vi "Rotating_Array.vi"() -> ()   [LabVIEW 2024]
panel:
  out "array (last n elements first)":dbl[](array[numeric])
  out "Array":sgl[](array[numeric])
  in  "Numeric":i32
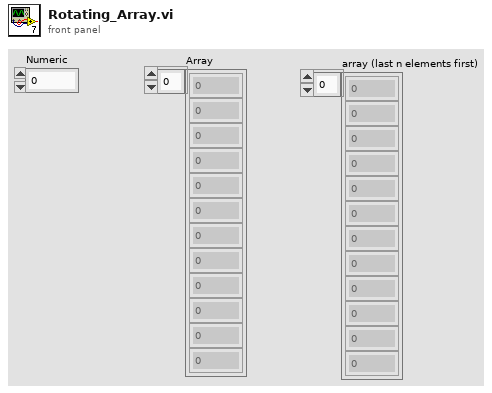
[diagram p1: front panel]
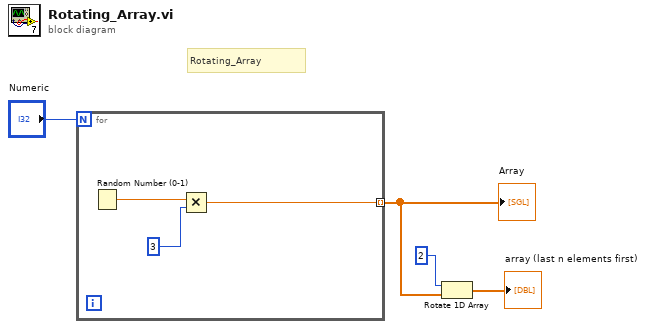
[diagram p0: block diagram]
diagram:
  # "Rotating_Array"
  n1 = for {
    N: "Numeric" -> [_]
    tunnel: [w5] -> w3 mode=indexing
    n2 = Random Number (0-1)() -> (number: 0 to 1=w7:dbl)
    n3 = Multiply(x=w7, y=3) -> (x*y=w5:dbl)
  }
  "Array" <- w3
  n4 = Rotate 1D Array(1:w3, 2:2 ("n")) -> (0:→"array (last n elements first)":dbl[])
